vi "SerialRead&Send.vi"(2 "写入配置":cluster{"命令":string, "是否写入":bool}={"命令"="*IDN?", "是否写入"=FALSE}, 3 "VISA resource name in":refnum<visa-resource-name>) -> (0 "响应":string, 1 "VISA resource name out":refnum<visa-resource-name>)   [LabVIEW 2019]
panel:
  out "返回数":u32
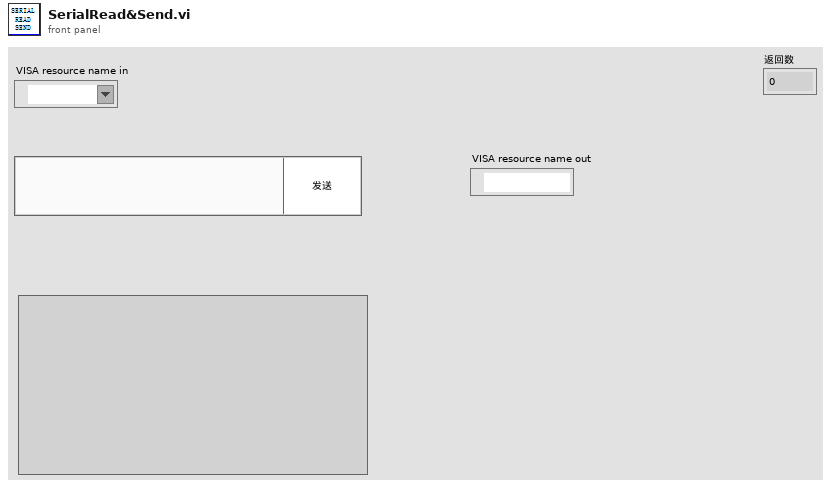
[diagram p1: front panel]
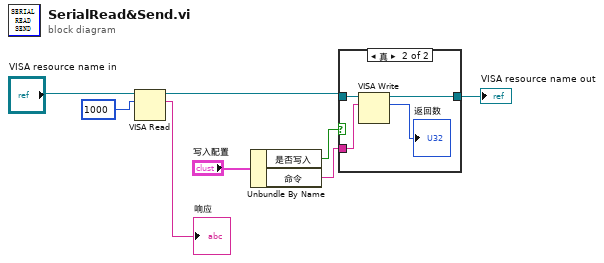
[diagram p0: block diagram]
diagram:
  n1 = VISA Read(VISA resource name="VISA resource name in", byte count=u32 1000 ("字节总数")) -> (VISA resource name out=w2:refnum<visa-resource-name>, read buffer=→"响应":string)  [unwired: 1 in, 2 out]
  n2 = Unbundle By Name("写入配置") -> ("是否写入"=w5:bool, "命令"=w7:string)
  n3 = case shown="真" w5 {
    tunnel: w2 -> [w9 w13]
    tunnel: [w9 w12] -> w6
    tunnel: w7 -> [_ w11]
    frame False {
    }
    frame True {
      n4 = VISA Write(VISA resource name=w13, write buffer=w11) -> (VISA resource name out=w12:refnum<visa-resource-name>, return count=→"返回数":u32)  [unwired: 1 in, 1 out]
    }
  }
  "VISA resource name out" <- w6
